vi "Write data.vi"(8 "error in":errorcluster, 10 "data":variant, 11 "communicator message in":refnum<class "communicator message.lvclass">) -> (0 "error out":errorcluster, 3 "communicator message out":refnum<class "communicator message.lvclass">)   [LabVIEW 2015]
uses:
  communicator message.lvclass
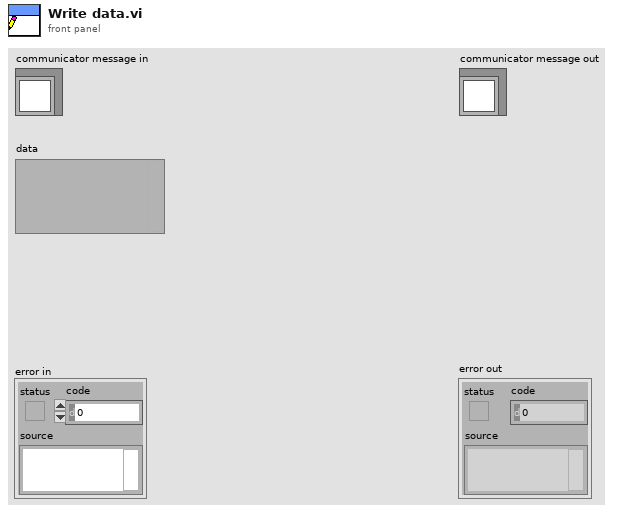
[diagram p1: front panel]
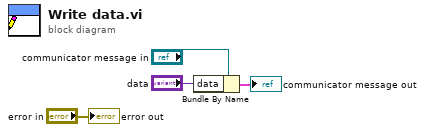
[diagram p0: block diagram]
diagram:
  n1 = Bundle By Name(cluster="communicator message in", "data"="data") -> (→"communicator message out":cluster{})
  "error out" <- "error in"
